vi "Loop_ACT_Solenoid.vi"() -> ()   [LabVIEW 2017, in "Claw.lvlib"]
uses:
  Claw.lvlib
  <vilib>/Rock Robotics/WPI/Solenoid/WPI_SolenoidValue.ctl
  Globals/Global_Device_IDs.vi
  <vilib>/Rock Robotics/WPI/Solenoid/WPI_SolenoidOpenDouble.vi
  _SHARE ALL/Global Share All/Global_STOP.vi
  Global_SM Write_Data Out.vi
  <vilib>/Rock Robotics/WPI/Solenoid/WPI_SolenoidSetEnum.vi
  <vilib>/Rock Robotics/WPI/Solenoid/WPI_SolenoidGetEnum.vi
  Global_ACT Write_Data Out.vi
panel:
  out "Solonoid Output":T1
  out "Cycle Time (S)":dbl format="%.3g"
  in  "Target Time(ms)":u32=50
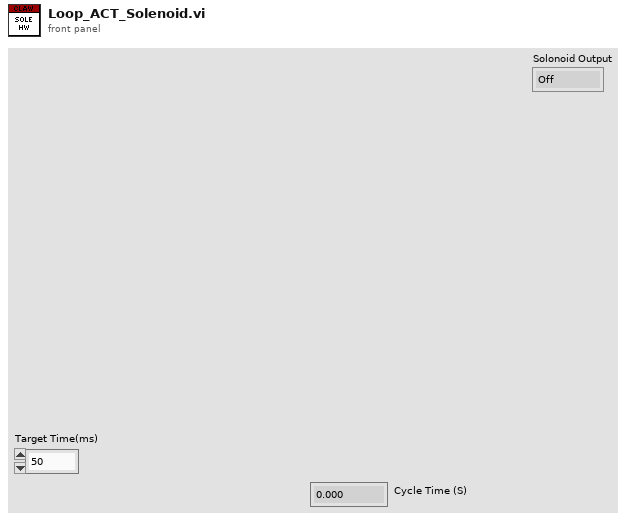
[diagram p1: front panel]
types:
  T1 = typedef "WPI_SolenoidValue.ctl" = enum16{"Off", "On", "Forward", "Reverse"}
  T2 = typedef "CLUSTER_Claw_Setup.ctl" = cluster{"Left Motor Setup":T3, "Right Motor Setup":T3, "Left Motor PDP":i32, "Right Motor PDP":i32, "Solonoid Setup":T5, "Limit Switch DIO":T7}
  T3 = typedef "CLUSTER_PWM Motor Setup.ctl" = cluster{"Motor PWM":T4, "Invert Motor":bool}
  T4 = typedef "FPGA_DIOPWMChannel.ctl" = enum8{"PWM 0", "PWM 1", "PWM 2", "PWM 3", "PWM 4", "PWM 5", "PWM 6", "PWM 7", "PWM 8", "PWM 9", "PWM MXP 0", "PWM MXP 1", "PWM MXP 2", "PWM MXP 3", "PWM MXP 4", "PWM MXP 5", "PWM MXP 6", "PWM MXP 7", "PWM MXP 8", "PWM MXP 9", "Invalid"}
  T5 = typedef "CLUSTER_Solonoid_Setup.ctl" = cluster{"Pneumatics Control Module (0)":u8, "Forward Solenoid Channel":T6, "Reverse Solenoid Channel":T6}
  T6 = typedef "WPI_SolenoidChannel.ctl" = enum8{"Solenoid 0", "Solenoid 1", "Solenoid 2", "Solenoid 3", "Solenoid 4", "Solenoid 5", "Solenoid 6", "Solenoid 7", "Invalid"}
  T7 = typedef "FPGA_DIOChannel.ctl" = enum8{"DIO 0", "DIO 1", "DIO 2", "DIO 3", "DIO 4", "DIO 5", "DIO 6", "DIO 7", "DIO 8", "DIO 9", "DIO MXP 0", "DIO MXP 1", "DIO MXP 2", "DIO MXP 3", "DIO MXP 4", "DIO MXP 5", "DIO MXP 6", "DIO MXP 7", "DIO MXP 8", "DIO MXP 9", "DIO MXP 10", "DIO MXP 11", "DIO MXP 12", "DIO MXP 13", "DIO MXP 14", "DIO MXP 15", "SPI Port CS1", "SPI Port CS2", "SPI Port CS3", "SPI Port MISO", "SPI Port MOSI", "Invalid"}
  T8 = typedef "WPI_SolenoidDevRef.ctl" = cluster{"DevStatus":errorcluster, "Pneumatics Control Module":u8, "Forward Solenoid Channel":T6, "Reverse Solenoid Channel":T6}
  T9 = cluster{"SolenoidDevRef":T8, "Solonoid Input":T1, "Solonoid Output":T1, "Target Time(ms)":u32, "Current Time":timestamp, "Previous Time":timestamp, "Cycle Time (S)":dbl}
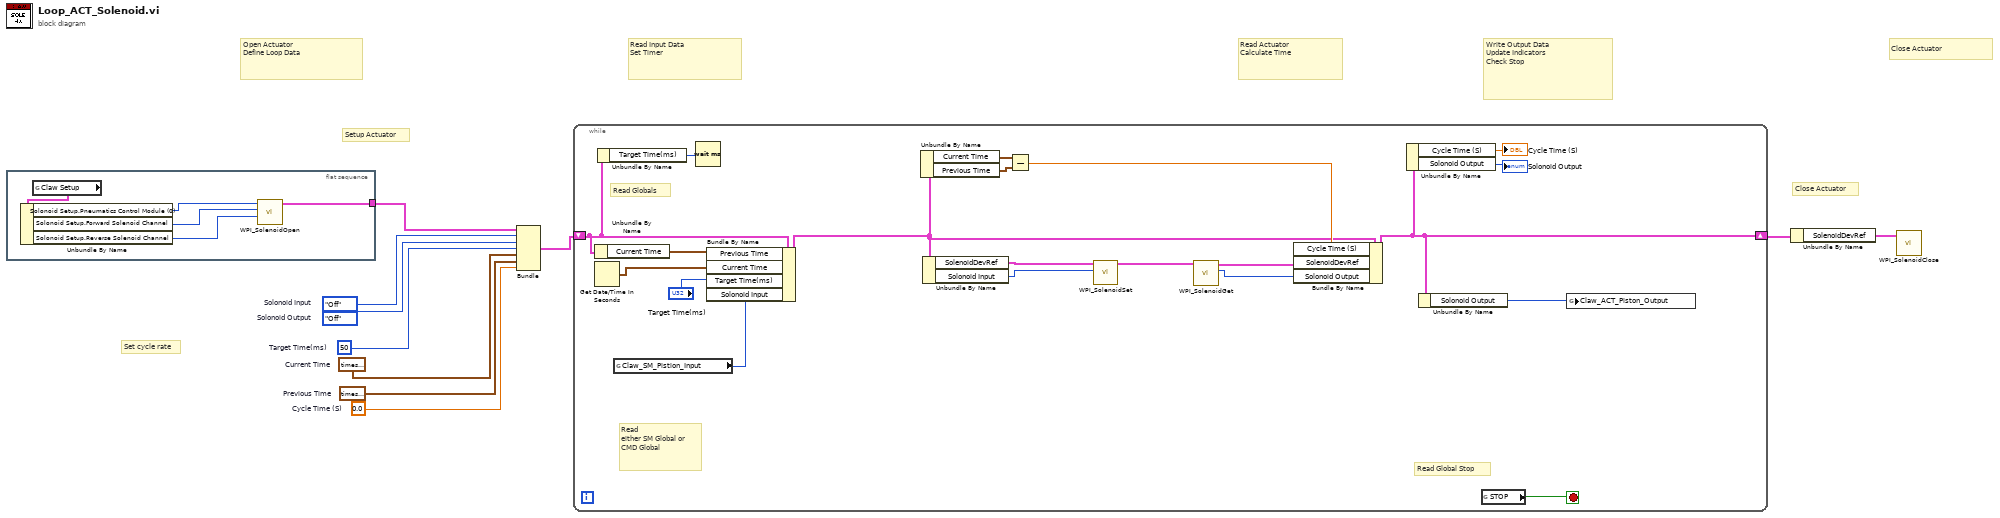
[diagram p0: block diagram]
diagram:
  w2 = WPI_SolenoidValue."Off"  # Solonoid Output
  w3 = WPI_SolenoidValue."Off"  # Solonoid Input
  w5 = 0.0  # Cycle Time (S)
  w10 = timestamp(0 s since 1904-01-01)  # Previous Time
  w9 = timestamp(0 s since 1904-01-01)  # Current Time
  w8 = u32 50  # Target Time(ms)
  # "Close Actuator"
  # "Write Output Data\nUpdate Indicators\nCheck Stop"
  # "Read Actuator\nCalculate Time"
  # "Read Input Data\nSet Timer"
  # "Open Actuator\nDefine Loop Data"
  # "Set cycle rate"
  # "Close Actuator"
  # "Setup Actuator"
  n1 = flat-sequence {
    tunnel: [w14] -> w4
    frame #0 {
      n2 = global read "Global_Device_IDs.vi" "Claw Setup"() -> (w15:T2)
      n3 = Unbundle By Name(w15) -> ("Solonoid Setup.Pneumatics Control Module (0)"=w13:u8, "Solonoid Setup.Forward Solenoid Channel"=w12:T6, "Solonoid Setup.Reverse Solenoid Channel"=w11:T6)
      n4 = call-poly <vilib>:"WPI_SolenoidOpen.vi"("Reverse Solenoid Channel"=w11, "Forward Solenoid Channel"=w12, "Pneumatics Control Module (0)"=w13) -> ("SolenoidDevRef"=w14:T8)  [unwired: 7 in, 1 out]
    }
  }
  n5 = Bundle("SolenoidDevRef"=w4, "Solonoid Input"=w3, "Solonoid Output"=w2, "Target Time(ms)"=w8, "Current Time"=w9, "Previous Time"=w10, "Cycle Time (S)"=w5) -> (w7:T9)  [unwired: 1 in]
  n6 = while {
    shift-right: [w27] -> w6
    shift-left: w7 -> [w29]
    stop <- w35 stop-if-true
    # "Read\neither SM Global or CMD Global"
    # "Read Globals"
    # "Read Global Stop"
    n7 = Unbundle By Name(w29) -> ("Current Time"=w33:timestamp)
    n8 = Get Date/Time In Seconds() -> (seconds since 1Jan1904=w34:timestamp)
    n9 = Unbundle By Name(w29) -> ("Target Time(ms)"=w28:u32)
    n10 = global read "Global_SM Write_Data Out.vi" "Claw_SM_Pistion_Input"() -> (w20:T1)
    n11 = Wait (ms)(milliseconds to wait=w28) -> ()  [unwired: 1 out]
    n12 = Bundle By Name(cluster=w29, "Previous Time"=w33, "Current Time"=w34, "Target Time(ms)"="Target Time(ms)", "Solonoid Input"=w20) -> (w24:T9)
    n13 = Unbundle By Name(w24) -> ("Current Time"=w32:timestamp, "Previous Time"=w31:timestamp)
    n14 = Unbundle By Name(w24) -> ("SolenoidDevRef"=w23:T8, "Solonoid Input"=w19:T1)
    n15 = Subtract(x=w32, y=w31) -> (x-y=w25:dbl)
    n16 = call-poly <vilib>:"WPI_SolenoidSet.vi"("Value"=w19, "SolenoidDevRef"=w23) -> ("SolenoidDevRef"=w22:T8)  [unwired: 8 in, 1 out]
    n17 = call-poly <vilib>:"WPI_SolenoidGet.vi"("SolenoidDevRef"=w22) -> ("Value"=w18:T1, "SolenoidDevRef"=w21:T8)  [unwired: 8 in, 1 out]
    n18 = Bundle By Name(cluster=w24, "Cycle Time (S)"=w25, "SolenoidDevRef"=w21, "Solonoid Output"=w18) -> (w27:T9)
    n19 = Unbundle By Name(w27) -> ("Cycle Time (S)"=→"Cycle Time (S)":dbl, "Solonoid Output"=→"Solonoid Output":T1)
    n20 = Unbundle By Name(w27) -> ("Solonoid Output"=w17:T1)
    n21 = global read "Global_STOP.vi" "STOP"() -> (w35:bool)
    n22 = global write "Global_ACT Write_Data Out.vi" "Claw_ACT_Piston_Output"(w17) -> ()
  }
  n23 = Unbundle By Name(w6) -> ("SolenoidDevRef"=w1:T8)
  n24 = call <vilib>:"WPI_SolenoidClose.vi"("SolenoidDevRef"=w1) -> ()  [unwired: 10 in, 1 out]
